vi "Refresh Instruments List.vi"(7 "UI Ref":refnum<vi>, 8 "error in (no error)":errorcluster, 9 "NewVal":i32, 10 "VerticalPicTextList Refnum":refnum<vi>, 11 "StoreUI in":refnum<class "StoreUI.lvclass">) -> (0 "error out":errorcluster, 3 "StoreUI out":refnum<class "StoreUI.lvclass">)   [LabVIEW 2015, in "StoreUI.lvlib" / "StoreUI.lvclass"]
uses:
  StoreUI.lvclass
  <userlib>/_XDesign Controls/VerticalPicTextList XControl/VerticalPicTextList.xctl
  StoreUI.lvclass/StoreUI.ctl
  VI Store/VIStore Actor/VIStore.lvclass/VIStore.ctl
  Classes/Category/Category.lvclass/Category.ctl
  Classes/Category/Category.lvclass
  Classes/Generic Item/Generic Item.lvclass
  VI Store/VIStore Actor/VIStore.lvclass
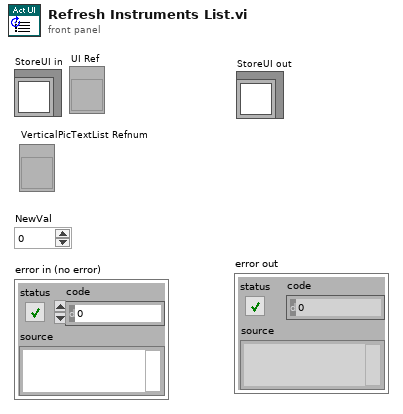
[diagram p1: front panel]
types:
  T1 = typedef "imagedata.ctl" = cluster{"image type":i32, "image depth":i32, "image":u8[], "mask":u8[], "colors":u32[], "Rectangle":cluster{"left":i16, "top":i16, "right":i16, "bottom":i16}}
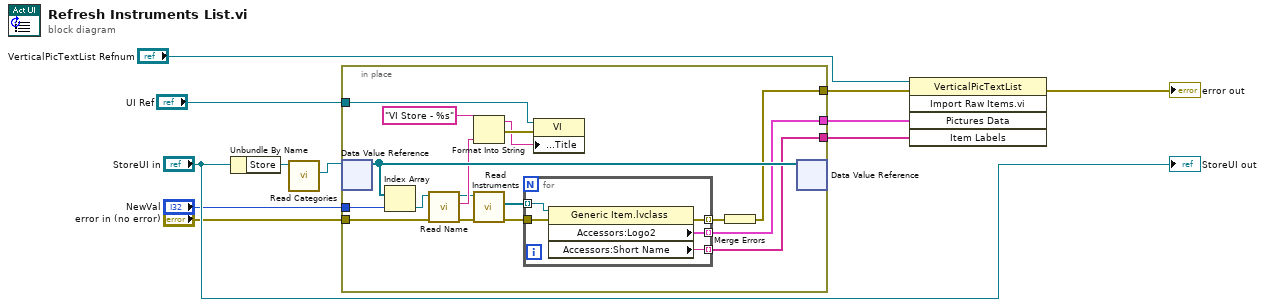
[diagram p0: block diagram]
diagram:
  n1 = Unbundle By Name("StoreUI in") -> ("Store"=w2:refnum<class "VIStore.lvclass">)
  n2 = call "Read Categories.vi"("VIStore in"=w2) -> ("Categories"=w1:refnum<data-value>)  [unwired: 8 in, 2 out]
  n3 = in-place {
    in-place-border: "NewVal" -> [w28]
    in-place-border: [w25] -> w4
    in-place-border: [w24] -> w3
    in-place-border: "error in (no error)" -> [w17]
    in-place-border: [w21] -> w5
    in-place-border: "UI Ref" -> [w13]
    n4 = in-place-dvr #1(w1) -> (w26:refnum<class "Category.lvclass">[])  [unwired: 1 out]
    n5 = Index Array(array=w26, index=w28) -> (element=w16:refnum<class "Category.lvclass">)
    n6 = call "Read Name.vi"("error in (no error)"=w17, "Category in"=w16) -> ("error out"=w14:errorcluster, "Name"=w18:string, "Category out"=w15:refnum<class "Category.lvclass">)  [unwired: 7 in]
    n7 = Format Into String(format string="VI Store - %s", w18) -> (resulting string=w12:string, error out=w20:errorcluster)  [unwired: 2 in]
    n8 = call-dynamic "Read Instruments.vi"("error in (no error)"=w14, "Category in"=w15) -> ("error out"=w23:errorcluster, "Instruments"=w27:refnum<class "Generic Item.lvclass">[])  [unwired: 7 in, 1 out]
    n9 = for {
      tunnel: w27 -> [w33] mode=indexing
      tunnel: [w32] -> w25 mode=indexing
      tunnel: [w31] -> w24 mode=indexing
      tunnel: w23 -> [w30]
      tunnel: [w29] -> w22 mode=indexing
      n10 = property class="Generic Item.lvclass"(reference=w33, error in=w30) -> (error out=w29:errorcluster, "Accessors:Logo2"=w32:T1, "Accessors:Short Name"=w31:string)  [unwired: 1 out]
    }
    n11 = property class="VI"(reference=w13, error in=w20, "Front Panel.Title"=w12) -> ()  [unwired: 2 out]
    n12 = Merge Errors(w22) -> (w21:errorcluster)
    n13 = in-place-dvr #1(w26) -> ()  [unwired: 2 out]
  }
  n14 = invoke class="VerticalPicTextList" method="Import Raw Items.vi"(reference="VerticalPicTextList Refnum", error in=w5, "Pictures Data"=w4, "Item Labels"=w3) -> (error out=→"error out":errorcluster)  [unwired: 1 in, 4 out]
  "StoreUI out" <- "StoreUI in"
